vi "MC5e Add_to_Q.vi"(5 "Priority":bool, 7 "queue":refnum<queue>, 8 "Error In":errorcluster, 9 "Variant":variant, 10 "Data":string, 11 "Command":string) -> (0 "error out":errorcluster, 3 "queue out":refnum<queue>)   [LabVIEW 2020]
uses:
  MC5e Command Q.ctl
  MC5e Gobal_Variables.vi
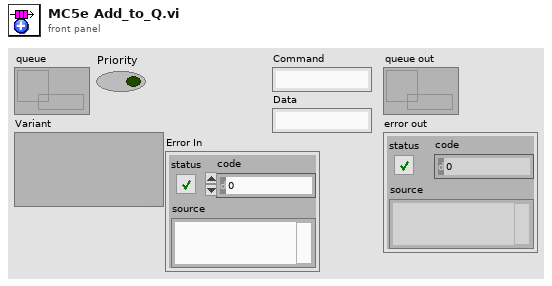
[diagram p1: front panel]
types:
  T1 = typedef "MC5e Command Q.ctl" = cluster{"Command":string, "Data String":string, "Variant":variant}
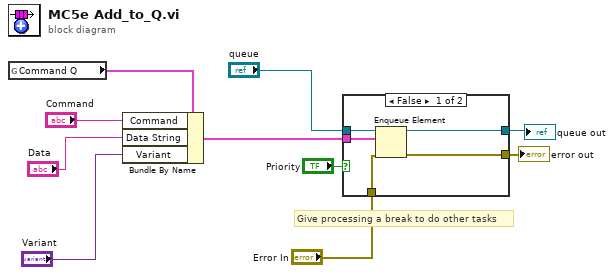
[diagram p0: block diagram]
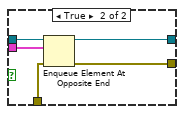
[diagram p2: hidden frame]
diagram:
  # "Give processing a break to do other tasks"
  n1 = global read "MC5e Gobal_Variables.vi" "Command Q"() -> (w8:T1)
  n2 = Bundle By Name(cluster=w8, "Command"="Command", "Data String"="Data", "Variant"="Variant") -> (w7:T1)
  n3 = case shown="False" "Priority" {
    tunnel: w7 -> [w15 w19]
    tunnel: "queue" -> [w14 w20]
    tunnel: [w13 w18] -> w3
    tunnel: [w12 w17] -> w2
    tunnel: "Error In" -> [w11 w16]
    frame False {
      n4 = Enqueue Element(queue=w14, element=w15, error in (no error)=w11) -> (queue out=w13:refnum<queue>, error out=w12:errorcluster)  [unwired: 1 in, 1 out]
    }
    frame True {
      n5 = Enqueue Element At Opposite End(queue=w20, element=w19, error in (no error)=w16) -> (queue out=w18:refnum<queue>, error out=w17:errorcluster)  [unwired: 1 in, 1 out]
    }
  }
  "queue out" <- w3
  "error out" <- w2
